vi "GPS change v3.vi"(8 "Angle":i16, 9 "Change":cluster{"X":dbl, "Y":dbl}, 11 "GPS in":cluster{"X":dbl, "Y":dbl}={"X"=1660.0, "Y"=340.0}) -> (3 "GPS out":cluster{"X":dbl, "Y":dbl})   [LabVIEW 2020]
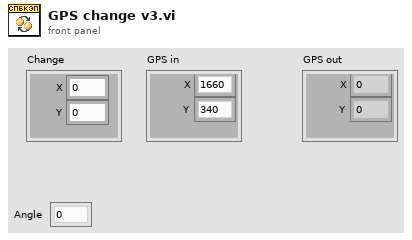
[diagram p1: front panel]
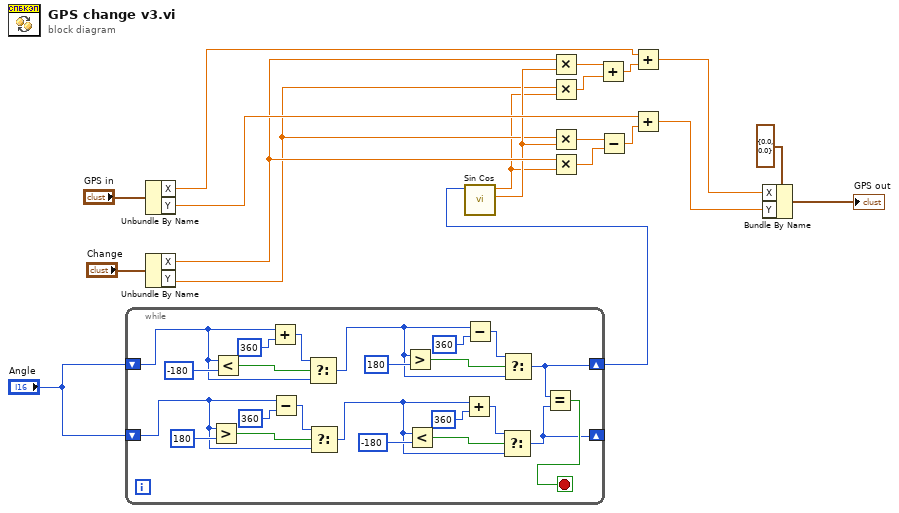
[diagram p0: block diagram]
diagram:
  n1 = while {
    shift-right: [w21] -> _
    shift-left: "Angle" -> [w39]
    shift-right: [w22] -> w2
    shift-left: "Angle" -> [w33]
    stop <- w36 stop-if-true
    n2 = Greater?(x=w39, y=i16 180) -> (0:w42:bool)
    n3 = Less?(x=w33, y=i16 -180) -> (x < y?=w35:bool)
    n4 = Add(x=w33, y=i16 360) -> (x+y=w37:i16)
    n5 = Subtract(x=w39, y=i16 360) -> (x-y=w43:i16)
    n6 = Select(t=w37, s=w35, f=w33) -> (s? t:f=w24:i16)
    n7 = Select(t=w43, s=w42, f=w39) -> (s? t:f=w23:i16)
    n8 = Greater?(x=w24, y=i16 180) -> (0:w30:bool)
    n9 = Less?(x=w23, y=i16 -180) -> (x < y?=w27:bool)
    n10 = Add(x=w23, y=i16 360) -> (x+y=w26:i16)
    n11 = Subtract(x=w24, y=i16 360) -> (x-y=w29:i16)
    n12 = Select(t=w26, s=w27, f=w23) -> (s? t:f=w21:i16)
    n13 = Select(t=w29, s=w30, f=w24) -> (s? t:f=w22:i16)
    n14 = Equal?(x=w22, y=w21) -> (x = y?=w36:bool)
  }
  n15 = Unbundle By Name("GPS in") -> ("X"=w7:dbl, "Y"=w18:dbl)
  n16 = Unbundle By Name("Change") -> ("X"=w14:dbl, "Y"=w4:dbl)
  n17 = call "Sin Cos.vi"("Angle"=w2) -> ("Cos"=w12:dbl, "Sin"=w3:dbl)  [unwired: 9 in]
  n18 = Multiply(x=w14, y=w12) -> (x*y=w6:dbl)
  n19 = Multiply(x=w4, y=w3) -> (x*y=w5:dbl)
  n20 = Multiply(x=w4, y=w12) -> (x*y=w15:dbl)
  n21 = Multiply(x=w14, y=w3) -> (x*y=w16:dbl)
  n22 = Add(x=w6, y=w5) -> (x+y=w8:dbl)
  n23 = Subtract(x=w15, y=w16) -> (x-y=w17:dbl)
  n24 = Add(x=w7, y=w8) -> (x+y=w9:dbl)
  n25 = Add(x=w18, y=w17) -> (x+y=w13:dbl)
  n26 = Bundle By Name(cluster=cluster{"X":dbl, "Y":dbl} {"X"=0.0, "Y"=0.0} ("GPS out"), "X"=w9, "Y"=w13) -> (→"GPS out":cluster{"X":dbl, "Y":dbl})
